vi "Delete Category.vi"(8 "error in (no error)":errorcluster, 10 "Category Name":string, 11 "Budgetizer in":refnum<class "Budgetizer.lvclass">) -> (0 "error out":errorcluster, 2 "Anything Deleted?":bool, 3 "Budgetizer out":refnum<class "Budgetizer.lvclass">)   [LabVIEW 2018, in "Budgetizer.lvclass"]
uses:
  Budgetizer.lvclass
  Budgetizer.lvclass/Budgetizer.ctl
  database/Database.lvclass
  Category/Category.lvclass
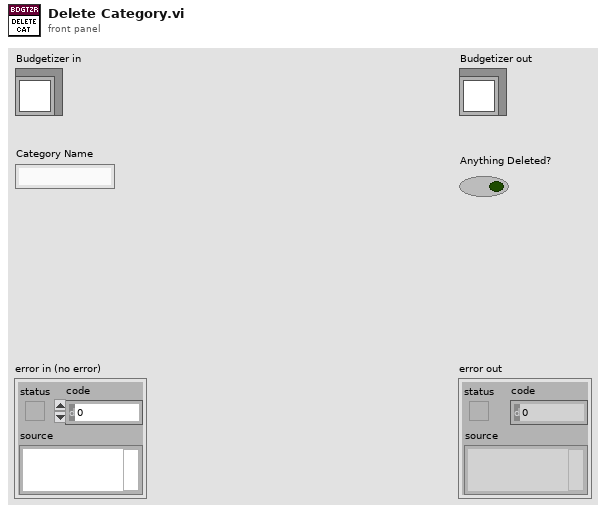
[diagram p1: front panel]
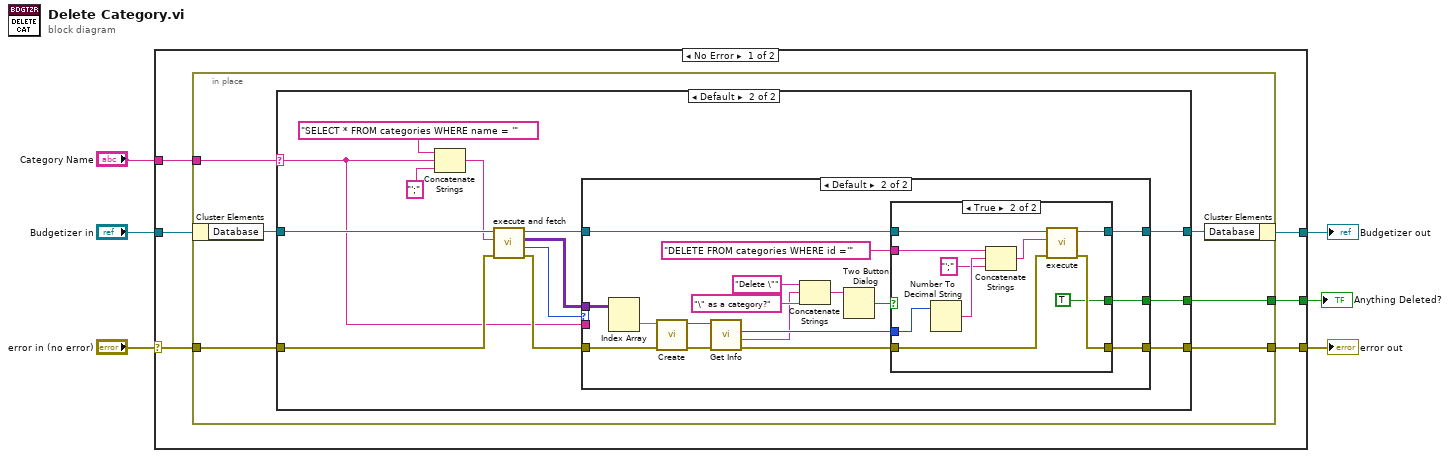
[diagram p0: block diagram]
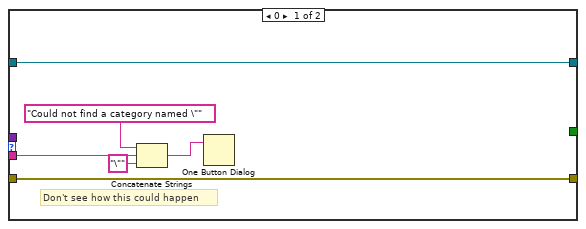
[diagram p3: hidden frame]
diagram:
  n1 = case shown="No Error" "error in (no error)" {
    selector: "error in (no error)" -> [w12 w70]
    tunnel: [w8 w70] -> w5
    tunnel: [w9 w69] -> w3
    tunnel: "Budgetizer in" -> [w11 w69]
    tunnel: "Category Name" -> [w10 _]
    tunnel: [w7 _] -> w1
    frame No Error {
      n2 = in-place {
        in-place-border: w12 -> [w17]
        in-place-border: w10 -> [w14]
        in-place-border: [w15] -> w8
        in-place-border: [w13] -> w7
        n3 = in-place-cluster #1(w11) -> ("Database"=w18:refnum<class "Database.lvclass">)
        n4 = case shown="Default" w14 {
          selector: w14 -> [_ w24]
          tunnel: w18 -> [w20 w33]
          tunnel: w17 -> [w19 w30]
          tunnel: [w20 w22] -> w16
          tunnel: [w19 w26] -> w15
          tunnel: [_ w21] -> w13
          frame "" {
          }
          frame Default {
            n5 = Concatenate Strings("SELECT * FROM categories WHERE name = '", w24, "';") -> (w29:string)
            n6 = call "execute and fetch.vi"("error in (no error)"=w30, "SQL query"=w29, "Database in"=w33) -> ("error out"=w27:errorcluster, "Num records"=w25:i32, "recordset data"=w28:variant[][], "Database out"=w23:refnum<class "Database.lvclass">)  [unwired: 5 in]
            n7 = case shown="Default" w25 {
              tunnel: w28 -> [_ w56]
              tunnel: w27 -> [w38 w54]
              tunnel: [w38 w44] -> w26
              tunnel: w24 -> [w39 _]
              tunnel: w23 -> [w34 w48]
              tunnel: [w34 w47] -> w22
              tunnel: [_ w42] -> w21
              frame 0 {
                # "Don't see how this could happen"
                n8 = Concatenate Strings("Could not find a category named \"", w39, "\"" ("string")) -> (w35:string)
                n9 = One Button Dialog(message=w35) -> ()  [unwired: 1 in, 1 out]
              }
              frame Default {
                n10 = Index Array(array=w56) -> (element=w55:variant[])  [unwired: 2 in]
                n11 = call "Create.vi"("error in (no error)"=w54, "Record"=w55) -> ("error out"=w52:errorcluster, "Category out"=w53:refnum<class "Category.lvclass">)  [unwired: 8 in]
                n12 = call "Get Info.vi"("error in (no error)"=w52, "Category in"=w53) -> ("error out"=w46:errorcluster, "Name"=w40:string, "id"=w41:i32)  [unwired: 6 in, 1 out]
                n13 = Concatenate Strings("Delete \"", w40, "\" as a category?" ("string")) -> (w49:string)
                n14 = Two Button Dialog(message=w49) -> (T button?=w45:bool)  [unwired: 2 in]
                n15 = case shown="True" w45 {
                  tunnel: w48 -> [w58 w68]
                  tunnel: [w58 w67] -> w47
                  tunnel: w46 -> [w57 w66]
                  tunnel: [w57 w65] -> w44
                  tunnel: w41 -> [_ w64]
                  tunnel: "DELETE FROM categories WHERE id ='" -> [_ w63]
                  tunnel: [_ TRUE ("Anything Deleted?")] -> w42
                  frame False {
                  }
                  frame True {
                    n16 = Number To Decimal String(number=w64) -> (decimal integer string=w61:string)  [unwired: 1 in]
                    n17 = Concatenate Strings(w63, w61, "';" ("string")) -> (w62:string)
                    n18 = call "execute.vi"("error in (no error)"=w66, "SQL query"=w62, "Database in"=w68) -> ("error out"=w65:errorcluster, "Database out"=w67:refnum<class "Database.lvclass">)  [unwired: 7 in]
                  }
                }
              }
            }
          }
        }
        n19 = in-place-cluster #1("Database"=w16) -> (w9:refnum<class "Budgetizer.lvclass">)
      }
    }
    frame Error {
    }
  }
  "error out" <- w5
  "Budgetizer out" <- w3
  "Anything Deleted?" <- w1
